vi "Read Full Force Test Settings.vi"(8 "error in (no error)":errorcluster, 11 "Boot Loader in":refnum<class "Boot Loader.lvclass">) -> (0 "error out":errorcluster, 2 "Full Force Test Settings":T1 {"SAA Force Set Points"."Axial Force" format="%.4f"; "SAA Force Set Points"."Lateral Force" format="%.4f"; "Max Moment (NM)" format="%.4f"; "Sample Time (s)" format="%.4f"; "Process Time (s)" format="%.4f"; "DAA Force Set Points"."Axial Force" format="%.4f"; "DAA Force Set Points"."Lateral Force" format="%.4f"; "Force Tolerance (N)" format="%.4f"}, 3 "Boot Loader out":refnum<class "Boot Loader.lvclass">)   [LabVIEW 2016]
uses:
  Boot Loader.lvclass
  Typedefs/FullForceScanSettings.ctl
  Typedefs/ForcePair.ctl
  Settings/Settings.lvclass
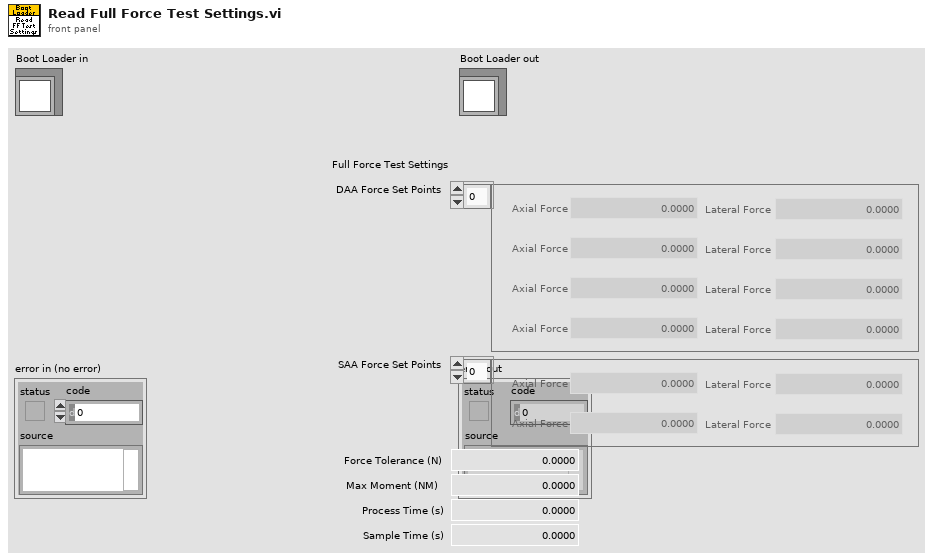
[diagram p1: front panel]
types:
  T1 = typedef "FullForceScanSettings.ctl" = cluster{"Force Tolerance (N)":dbl, "DAA Force Set Points":T2[], "Process Time (s)":dbl, "Sample Time (s)":dbl, "Max Moment (NM)":dbl, "SAA Force Set Points":T2[]}
  T2 = typedef "ForcePair.ctl" = cluster{"Axial Force":dbl, "Lateral Force":dbl}
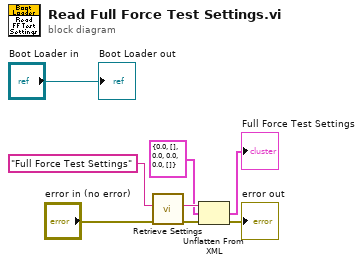
[diagram p0: block diagram]
diagram:
  n1 = call "Retrieve Settings.vi"("error in (no error)"="error in (no error)", "configName"="Full Force Test Settings") -> ("error out"=w4:errorcluster, "xmlConfig"=w7:string)  [unwired: 7 in, 1 out]
  n2 = Unflatten From XML(xml string=w7, type=T1 {"Force Tolerance (N)"=0.0, "DAA Force Set Points"=[], "Process Time (s)"=0.0, "Sample Time (s)"=0.0, "Max Moment (NM)"=0.0, "SAA Force Set Points"=[]} ("Full Force Test Settings"), error in (no error)=w4) -> (value=→"Full Force Test Settings":T1, error out=→"error out":errorcluster)
  "Boot Loader out" <- "Boot Loader in"
